vi "initVI.vi"() -> ()   [LabVIEW 2010]
panel:
  in  "VI引用句柄":refnum<vi>
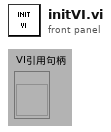
[diagram p1: front panel]
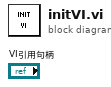
[diagram p0: block diagram]
diagram:
